vi "Tock7.vi"(1 "TimerRegisters":T1={"Tick0"="Tick0", "Tock0"="Tock0", "Tick1"="Tick1", "Tock1"="Tock1", "Tick2"="Tick1", "Tock2"="Tock1", "Tick3"="Tick1", "Tock3"="Tock1", "Tick4"="Tick0", "Tock4"="Tock0", "Tick5"="Tick1", "Tock5"="Tock1", "Tick6"="Tick1", "Tock6"="Tock1", "Tick7"="Tick1", "Tock7"="Tock1"}, 11 "valid input":bool) -> (15 "valid output":bool)   [LabVIEW 2015, in "Timers.lvlib"]
uses:
  Timers.lvlib
  TimerRegisters.ctl
  <vilib>/rvi/DataTransferAndStorage/Container/Common/niFpgaContainerExecOnDevCompGetState.vi
  <vilib>/rvi/Emulation/niFpgaEmulationIsFPGAContextNoSignature.vi
  <vilib>/rvi/DataTransferAndStorage/Container/Common/niFpgaContainerGetUniqueNameForEmu.vi
  <vilib>/rvi/Memory/Memory_Emulation/niFpgaMemoryEmulationCacheClearOnFirstRun.vi
  <vilib>/rvi/Memory/Memory_Emulation/nirvimemoryEmulationManagerCache_MakeExclusive.vi
  <vilib>/rvi/Memory/Memory_Emulation/niFpgaMemoryEmulationValidateCache.vi
  <vilib>/rvi/Memory/Memory_Emulation/nirvimemoryEmulationManagerCache_InsertValue.vi
  <vilib>/Utility/error.llb/Clear Errors.vi
  <vilib>/rvi/Memory/Memory_Emulation/nirvimemoryEmulationManagerCache_ReleaseExclusive.vi
  <vilib>/rvi/Memory/Memory_Emulation/nirvimemoryEmulationManagerCache_GetValue.vi
  <vilib>/rvi/Memory/Memory_Emulation/nirvimemoryEmulationManagerCache_SetValue.vi
  <vilib>/rvi/Emulation/niFpgaProcessEmulError.vi
  <vilib>/rvi/Emulation/niFpgaSctlEmulationGetInTimedLoop.vi
  <vilib>/rvi/DataTransferAndStorage/Container/XNode/niFpgaContainer.xnode
  <vilib>/rvi/DataTransferAndStorage/Register/Emulation/niFpgaRegisterEmulationRefIn.vi
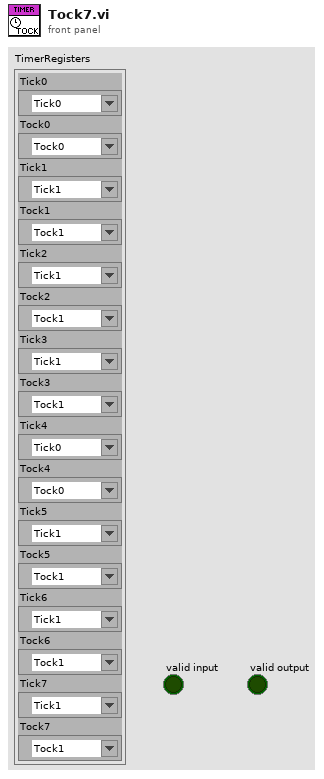
[diagram p1: front panel]
types:
  T1 = typedef "Timers.lvlib/TimerRegisters.ctl" = cluster{"Tick0":refnum<k21>, "Tock0":refnum<k21>, "Tick1":refnum<k21>, "Tock1":refnum<k21>, "Tick2":refnum<k21>, "Tock2":refnum<k21>, "Tick3":refnum<k21>, "Tock3":refnum<k21>, "Tick4":refnum<k21>, "Tock4":refnum<k21>, "Tick5":refnum<k21>, "Tock5":refnum<k21>, "Tick6":refnum<k21>, "Tock6":refnum<k21>, "Tick7":refnum<k21>, "Tock7":refnum<k21>}
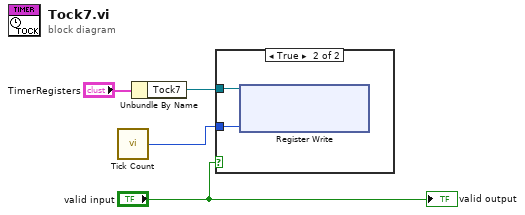
[diagram p0: block diagram]
diagram:
  n1 = call "Tick Count"() -> ("Tick Count(Ticks)"=w4:u32)
  n2 = Unbundle By Name("TimerRegisters") -> ("Tock7"=w1:refnum<k21>)
  n3 = case shown="True" "valid input" {
    tunnel: w1 -> [_ w6]
    tunnel: w4 -> [_ w5]
    frame False {
    }
    frame True {
      n4 = xnode ("Register Write")("Data"=w5, "Register In"=w6) -> ()  [unwired: 1 out]
    }
  }
  "valid output" <- "valid input"
